vi "psc_carrier_generator.vi"(9 "RST_in":bool, 10 "Step":u32=1, 11 "MAX":u32=1) -> (2 "PSC out":u32, 3 "RST_out":bool=TRUE)   [LabVIEW 2021]
doc: "This VI generates the next point on a DDS generated sine wave.\n\nThe accumulator increments to calculate the next phase value in the waveform. By varying the accumulator increment you control the frequency of the sine wave.\n\nThe accumulator phase value is used to select a value from the sine wave reference waveform stored in the Lookup Table VI. The waveformcan be p[hase shifted by specifying a non-zero phase shift value which is added to the accumulator phase. The output from the LUT is scaled using the AO Amplitude value."
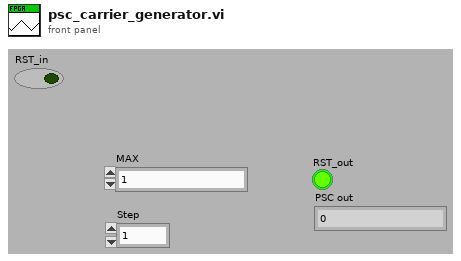
[diagram p1: front panel]
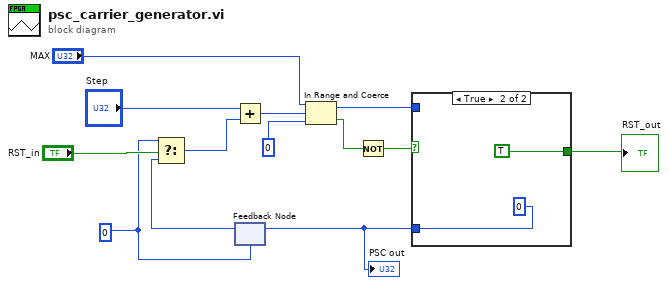
[diagram p0: block diagram]
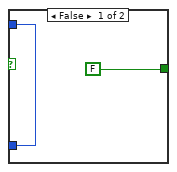
[diagram p2: hidden frame]
diagram:
  w5 = u32 0 ("x")
  n1 = feedback #1(w5) -> (w11:u32)
  n2 = Select(t=w5, s="RST_in", f=w11) -> (s? t:f=w4:u32)
  n3 = Add(x="Step", y=w4) -> (x+y=w2:u32)
  n4 = In Range and Coerce(upper limit="MAX", x=w2, lower limit=u32 0 ("x+y")) -> (coerced(x)=w12:u32, In Range?=w8:bool)
  n5 = Not(x=w8) -> (.not. x?=w9:bool)
  n6 = case shown="True" w9 {
    tunnel: [w15 u32 0 ("x+y")] -> w1
    tunnel: w12 -> [w15 _]
    tunnel: [FALSE TRUE] -> w10
    frame False {
    }
    frame True {
    }
  }
  "RST_out" <- w10
  "PSC out" <- w1
  n7 = feedback-in #1(w1) -> ()
